vi "Main NR.vi"(8 "error in":errorcluster, 11 "RT System Monitor in":refnum<class "RT System Monitor.lvclass">) -> (0 "error out":errorcluster, 3 "RT System Monitor out":refnum<class "RT System Monitor.lvclass">)   [LabVIEW 2017, in "RT System Monitor.lvclass"]
doc: "The <b>Queued Message Handler</b> of the Worker that owns this VI."
uses:
  RT System Monitor.lvclass
  Initialization Data.ctl
  Response Cases.ctl
  <vilib>/addons/_Workers/Library/Case Label.ctl
  RT System Monitor.lvclass/RT System Monitor.ctl
  rql_Initialize Session.ctl
  rql_Get System Properties.ctl
  rsp_Receive System Properties.ctl
  Shared/System Health Data.ctl
  <vilib>/nisyscfg/Close (Hardware).vi
  <vilib>/nisyscfg/Close (System).vi
  <vilib>/nisyscfg/nisyscfg.lvlib
  <resource>/objmgr/nisysapi.rc
  <vilib>/addons/_Workers/Library/Workers.lvlib
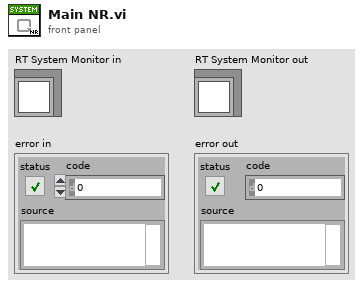
[diagram p1: front panel]
types:
  T1 = typedef "RT System Monitor.lvclass/Initialization Data.ctl" = cluster{"Response Cases":T2}
  T2 = typedef "RT System Monitor.lvclass/Response Cases.ctl" = cluster{"Receive System Properties":T3}
  T3 = typedef "Workers.lvlib/Case Label.ctl" = string
  T4 = typedef "RT System Monitor.lvclass/rql_Initialize Session.ctl" = cluster{"String":string}
  T5 = typedef "RT System Monitor.lvclass/rsp_Receive System Properties.ctl" = cluster{"System Health Data":T6}
  T6 = typedef "System Health Data.ctl" = cluster{"CPUs":u32[][], "Memory":dbl[][], "Hard Drive Space Used (%)":dbl, "Primary Hard Drive Available (MB)":dbl, "Primary Hard Drive Capacity (MB)":u32, "Total Physical Memory (MB)":u32, "Total Virtual Memory (MB)":u32}
  T7 = typedef "RT System Monitor.lvclass/rql_Get System Properties.ctl" = cluster{"String":string}
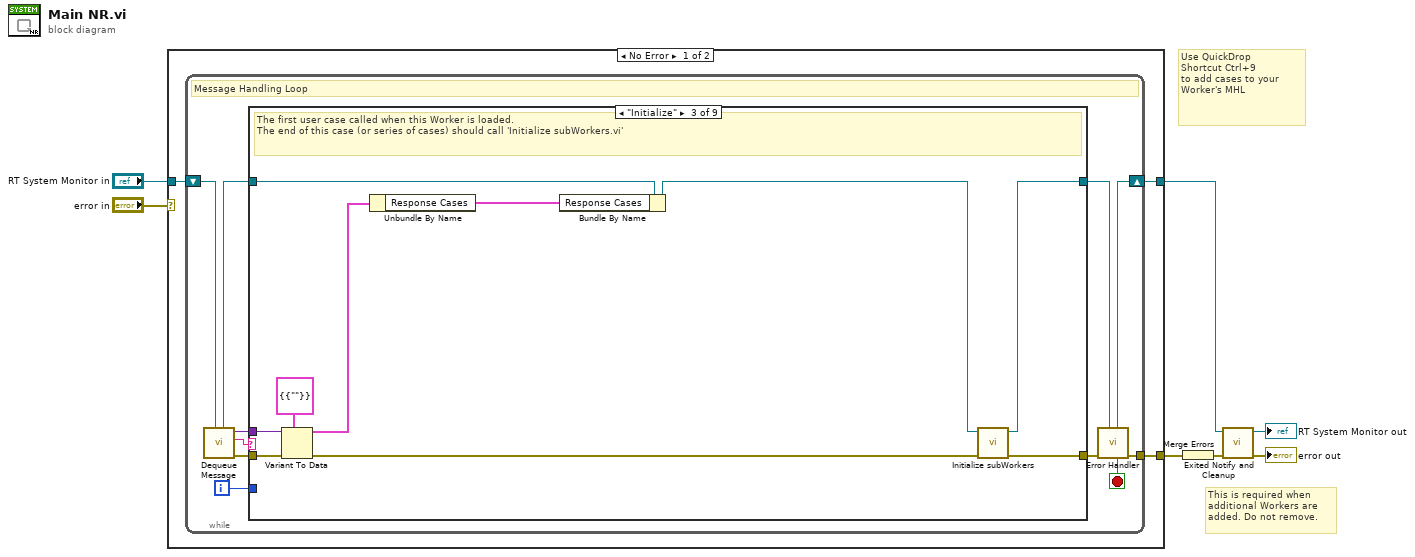
[diagram p0: block diagram]
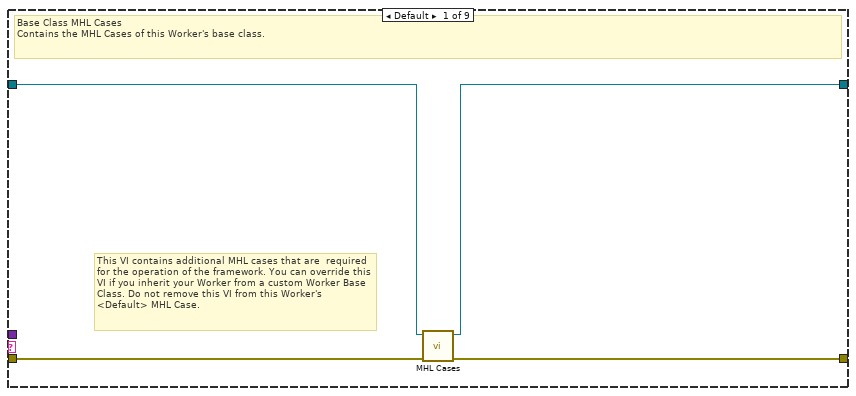
[diagram p2: hidden frame]
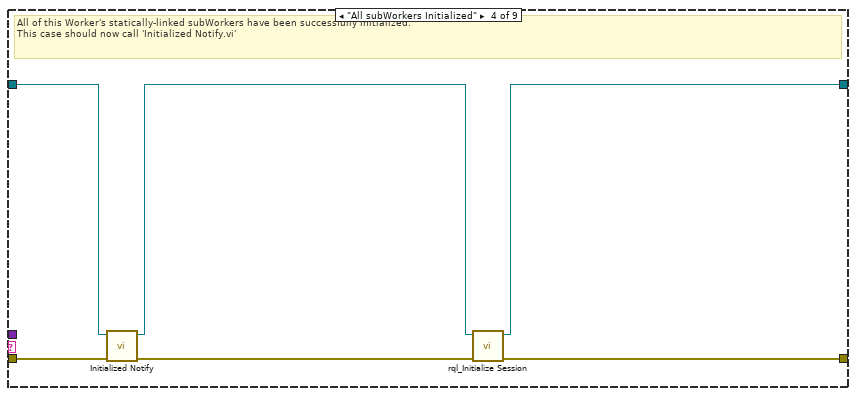
[diagram p4: hidden frame]
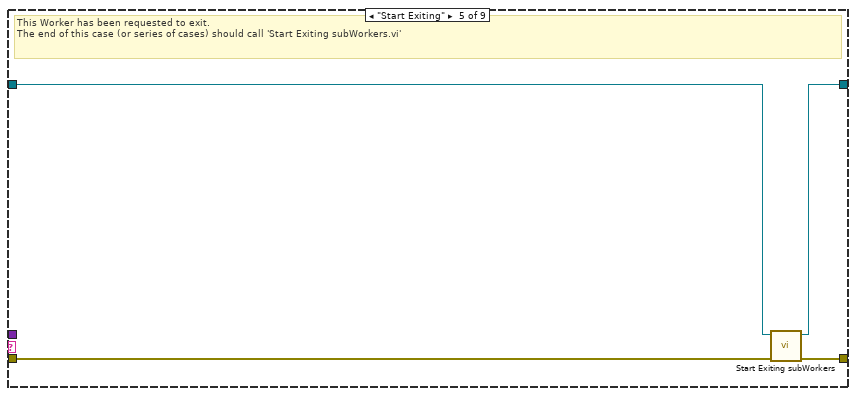
[diagram p5: hidden frame]
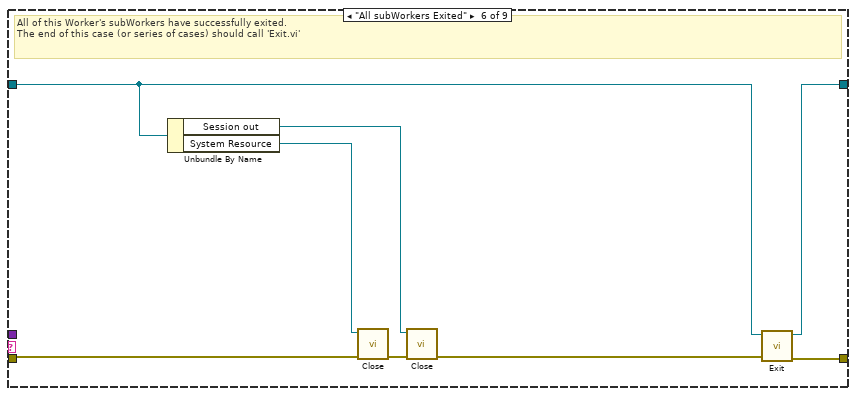
[diagram p6: hidden frame]
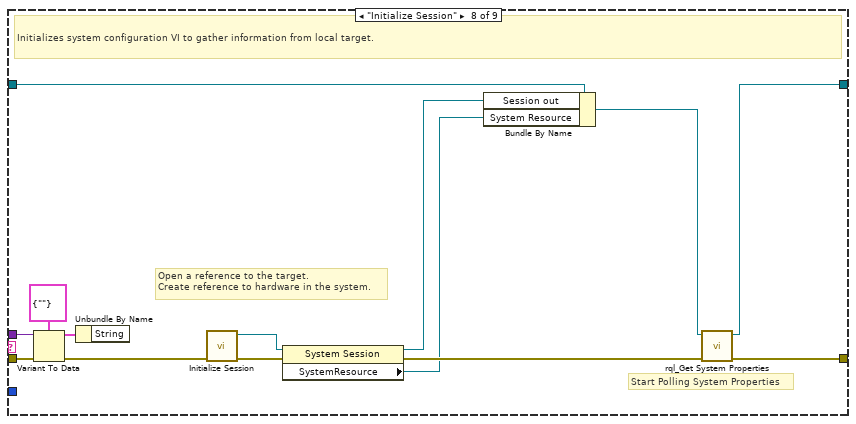
[diagram p8: hidden frame]
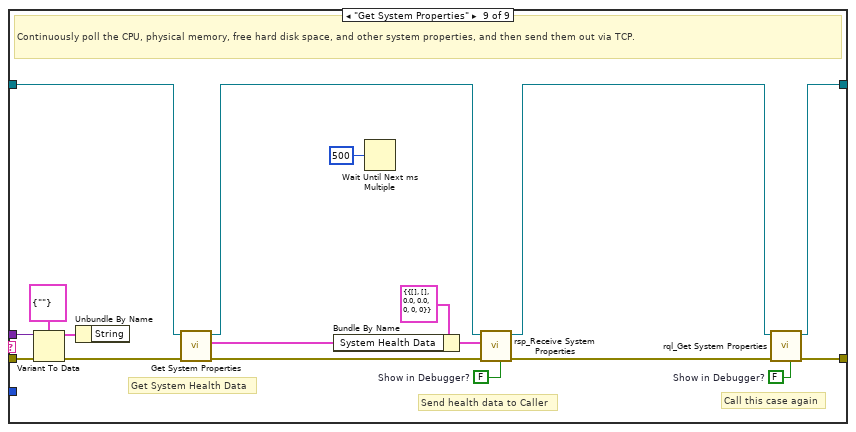
[diagram p9: hidden frame]
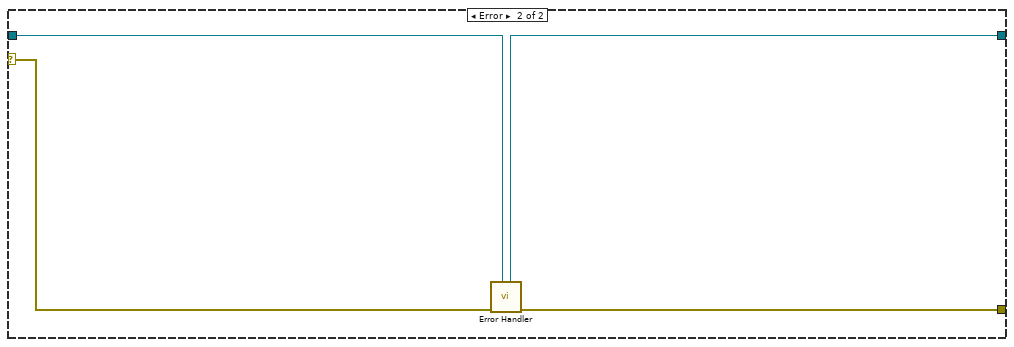
[diagram p10: hidden frame]
diagram:
  # "Use QuickDrop\nShortcut Ctrl+9\nto add cases to your\nWorker's MHL"
  # "This is required when additional Workers are added. Do not remove."
  n1 = case shown="No Error" "error in" {
    tunnel: "RT System Monitor in" -> [w8 w91]
    tunnel: [w10 w92] -> w6
    tunnel: [w9 w90] -> w7
    selector: "error in" -> [_ w93]
    frame No Error {
      n2 = while {
        shift-right: [w19] -> w9
        shift-left: w8 -> [w21]
        tunnel: [w20] -> w10
        i -> [w12]
        stop <- w13 stop-if-true
        # "Message Handling Loop"
        n3 = call-dynamic "Dequeue Message.vi"("Worker"=w21) -> ("error out"=w18:errorcluster, "Case out"=w14:string, "Data out"=w11:variant, "Worker out"=w16:refnum<class "RT System Monitor.lvclass">)  [unwired: 6 in, 1 out]
        n4 = case "Worker MHL Case Structure (DO NOT CHANGE LABEL NAME)" shown="\"Initialize\"" w14 {
          tunnel: w18 -> [w25 w26 w35 w43 w44 w52 w57 w70 w89]
          tunnel: [w24 w26 w37 w40 w47 w55 w57 w60 w82] -> w17
          tunnel: w16 -> [w23 w27 w30 w41 w45 w50 w56 w71 w84]
          tunnel: [w22 w27 w36 w38 w46 w54 w56 w58 w81] -> w15
          tunnel: w12 -> [_ _ _ _ _ _ _ _ _]
          tunnel: w11 -> [_ _ w33 _ _ _ _ w68 w86]
          frame Default {
            # "This VI contains additional MHL cases that are  required for the operation of the framework. You can override this VI if you inherit your Worker from a custom Worker Base Class. Do not remove this VI from this Worker's <Default> MHL Case."
            # "Base Class MHL Cases\nContains the MHL Cases of this Worker's base class."
            n5 = call-dynamic "MHL Cases.vi"("error in"=w25, "Worker in"=w23) -> ("error out"=w24:errorcluster, "Worker out"=w22:refnum<class "RT System Monitor.lvclass">)  [unwired: 8 in]
          }
          frame "------------ FRAMEWORK CASES -----------" {
            # "Start of Workers Framework Cases"
          }
          frame "Initialize" {
            # "The first user case called when this Worker is loaded.\nThe end of this case (or series of cases) should call 'Initialize subWorkers.vi'"
            n6 = Variant To Data(error in=w35, type=T1 {"Response Cases"={"Receive System Properties"=""}} ("Cluster"), Variant=w33) -> (data=w31:T1, error out=w34:errorcluster)
            n7 = Unbundle By Name(w31) -> ("Response Cases"=w32:T2)
            n8 = Bundle By Name(cluster=w30, "Response Cases"=w32) -> (w29:refnum<class "RT System Monitor.lvclass">)
            n9 = call-dynamic "Initialize subWorkers.vi"("error in"=w34, "Worker"=w29) -> ("error out"=w37:errorcluster, "dup Worker out"=w36:refnum<class "RT System Monitor.lvclass">)  [unwired: 8 in]
          }
          frame "All subWorkers Initialized" {
            # "All of this Worker's statically-linked subWorkers have been successfully initialized.\nThis case should now call 'Initialized Notify.vi'"
            n10 = call-dynamic "Initialized Notify.vi"("error in"=w43, "Worker"=w41) -> ("error out"=w42:errorcluster, "dup Worker out"=w39:refnum<class "RT System Monitor.lvclass">)  [unwired: 8 in]
            n11 = call "rql_Initialize Session.vi"("error in"=w42, "RT System Monitor in"=w39) -> ("error out"=w40:errorcluster, "dup RT System Monitor out"=w38:refnum<class "RT System Monitor.lvclass">)  [unwired: 8 in]
          }
          frame "Start Exiting" {
            # "This Worker has been requested to exit. \nThe end of this case (or series of cases) should call 'Start Exiting subWorkers.vi'"
            n12 = call-dynamic "Start Exiting subWorkers.vi"("error_in"=w44, "Worker"=w45) -> ("error out"=w47:errorcluster, "dup Worker out"=w46:refnum<class "RT System Monitor.lvclass">)  [unwired: 8 in]
          }
          frame "All subWorkers Exited" {
            # "All of this Worker's subWorkers have successfully exited. \nThe end of this case (or series of cases) should call 'Exit.vi'"
            n13 = Unbundle By Name(w50) -> ("Session out"=w49:refnum<k21>, "System Resource"=w48:refnum<k20>)
            n14 = call-poly <vilib>:"Close.vi"("error in (no error)"=w52, "Resource in"=w48) -> ("error out"=w53:errorcluster)  [unwired: 9 in]
            n15 = call-poly <vilib>:"Close.vi"("error in (no error)"=w53, "Session in"=w49) -> ("error out"=w51:errorcluster)  [unwired: 9 in]
            n16 = call-dynamic "Exit.vi"("error_in"=w51, "Worker"=w50) -> ("error out"=w55:errorcluster, "dup Worker out"=w54:refnum<class "RT System Monitor.lvclass">)  [unwired: 8 in]
          }
          frame "------------- LOCAL API CASES -------------" {
            # "Start of Workers Local API Cases"
          }
          frame "Initialize Session" {
            # "Start Polling System Properties"
            # "Open a reference to the target.\nCreate reference to hardware in the system."
            # "Initializes system configuration VI to gather information from local target."
            n17 = Variant To Data(error in=w70, type=T4 {"String"=""} ("Data"), Variant=w68) -> (data=w67:T4, error out=w65:errorcluster)
            n18 = Unbundle By Name(w67) -> ()  [unwired: 1 out]
            n19 = call <vilib>:"Initialize Session.vi"("error in (no error)"=w65) -> ("error out"=w66:errorcluster, "Session out"=w63:refnum<k21>)  [unwired: 9 in]
            n20 = property class="System Session"(reference=w63, error in=w66) -> (reference out=w62:refnum<k21>, error out=w64:errorcluster, "SystemResource"=w61:refnum<k20>)
            n21 = Bundle By Name(cluster=w71, "Session out"=w62, "System Resource"=w61) -> (w59:refnum<class "RT System Monitor.lvclass">)
            n22 = call "rql_Get System Properties.vi"("error in"=w64, "RT System Monitor in"=w59) -> ("error out"=w60:errorcluster, "dup RT System Monitor out"=w58:refnum<class "RT System Monitor.lvclass">)  [unwired: 8 in]
          }
          frame "Get System Properties" {
            w72 = FALSE  # Show in Debugger?
            w79 = FALSE  # Show in Debugger?
            # "Get System Health Data"
            # "Send health data to Caller"
            # "Call this case again"
            # "Continuously poll the CPU, physical memory, free hard disk space, and other system properties, and then send them out via TCP."
            n23 = Variant To Data(error in=w89, type=T7 {"String"=""} ("Data"), Variant=w86) -> (data=w85:T7, error out=w88:errorcluster)
            n24 = Unbundle By Name(w85) -> ()  [unwired: 1 out]
            n25 = call "Get System Properties.vi"("error in (no error)"=w88, "RT System Monitor in"=w84) -> ("error out"=w80:errorcluster, "System Health Data"=w73:T6, "RT System Monitor out"=w77:refnum<class "RT System Monitor.lvclass">)  [unwired: 7 in]
            n26 = Bundle By Name(cluster=T5 {"System Health Data"={"CPUs"=[], "Memory"=[], "Hard Drive Space Used (%)"=0.0, "Primary Hard Drive Available (MB)"=0.0, "Primary Hard Drive Capacity (MB)"=0, "Total Physical Memory (MB)"=0, "Total Virtual Memory (MB)"=0}} ("Data in"), "System Health Data"=w73) -> (w74:T5)
            n27 = Wait Until Next ms Multiple(millisecond multiple=u32 500 ("Polling Interval")) -> ()  [unwired: 1 out]
            n28 = call "rsp_Receive System Properties.vi"("Show in Debugger?"=w72, "error in"=w80, "Data in"=w74, "RT System Monitor in"=w77) -> ("error out"=w78:errorcluster, "dup RT System Monitor out"=w76:refnum<class "RT System Monitor.lvclass">)  [unwired: 6 in]
            n29 = call "rql_Get System Properties.vi"("Show in Debugger?"=w79, "error in"=w78, "RT System Monitor in"=w76) -> ("error out"=w82:errorcluster, "dup RT System Monitor out"=w81:refnum<class "RT System Monitor.lvclass">)  [unwired: 7 in]
          }
        }
        n30 = call-dynamic "Error Handler.vi"("Worker"=w15, "error_in"=w17) -> ("error out"=w20:errorcluster, "Stop Loop"=w13:bool, "Worker out"=w19:refnum<class "RT System Monitor.lvclass">)  [unwired: 7 in]
      }
    }
    frame Error {
      n31 = call-dynamic "Error Handler.vi"("Worker"=w91, "error_in"=w93) -> ("error out"=w92:errorcluster, "Worker out"=w90:refnum<class "RT System Monitor.lvclass">)  [unwired: 7 in, 1 out]
    }
  }
  n32 = Merge Errors(w6) -> (w3:errorcluster)
  n33 = call-dynamic "Exited Notify and Cleanup.vi"("error_in"=w3, "Worker"=w7) -> ("error out"=→"error out":errorcluster, "dup Worker out"=→"RT System Monitor out":refnum<class "RT System Monitor.lvclass">)  [unwired: 8 in]
